vi "Tray_Search_PressIndex.vi"(0 "TrayIn":refnum<vi>, 5 "XY_DTray":cluster{"X":i32, "Y":i32}={"X"=8, "Y"=16}, 7 "Press_Arr":bool[][](array[boolean]), 9 "Record_Arr In":bool[][](array[boolean])) -> (6 "Press_Arr Out":bool[][](array[boolean]), 8 "Record_Arr Out":bool[][](array[boolean]))   [LabVIEW 2019]
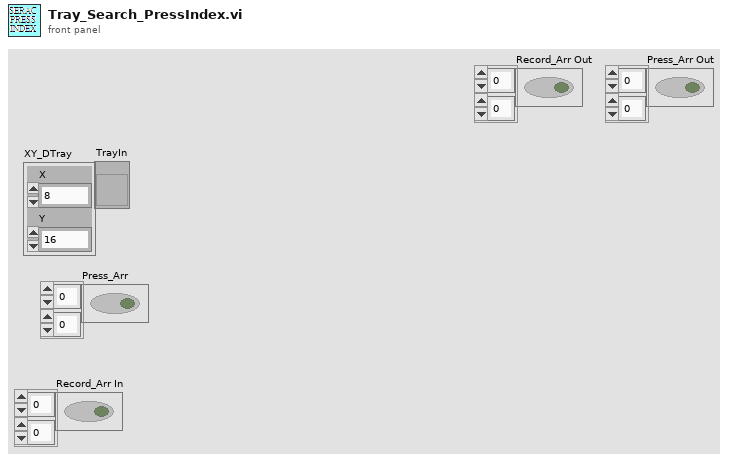
[diagram p1: front panel]
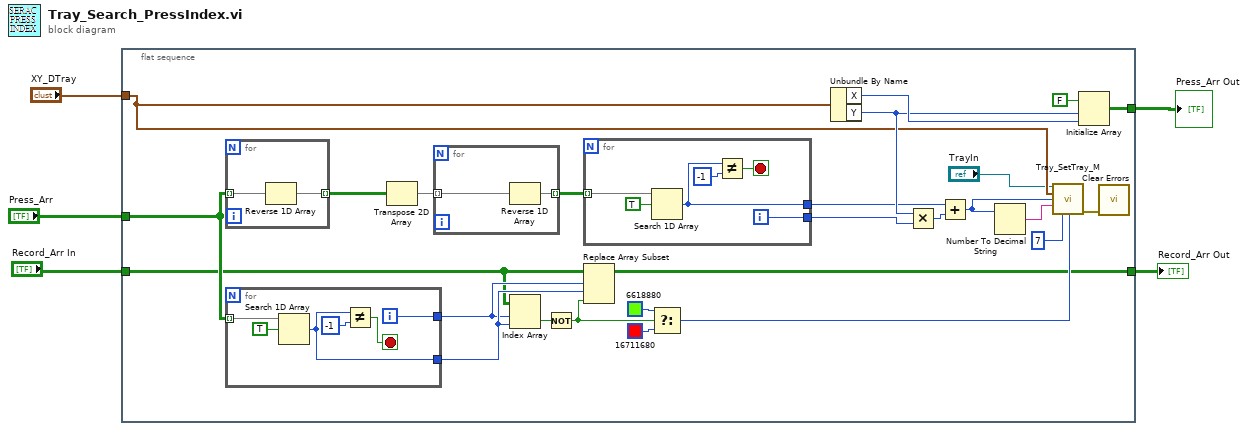
[diagram p0: block diagram]
diagram:
  n1 = flat-sequence {
    tunnel: [w26] -> w3
    tunnel: "Press_Arr" -> [w11]
    tunnel: "Record_Arr In" -> [w10]
    tunnel: "XY_DTray" -> [w9]
    tunnel: [w8] -> w1
    frame #0 {
      n2 = for {
        tunnel: [w47] -> w31 mode=indexing
        tunnel: w11 -> [w46] mode=indexing
        n3 = Reverse 1D Array(array=w46) -> (reversed array=w47:bool[])
      }
      n4 = for {
        tunnel: w11 -> [w37] mode=indexing
        tunnel: [w34] -> w12
        tunnel: [w33] -> w13
        i -> [w34]
        stop <- w35 stop-if-true
        n5 = Search 1D Array(1D array=w37, element=TRUE) -> (index of element=w33:i32)  [unwired: 1 in]
        n6 = Not Equal?(x=w33, y=-1) -> (x != y?=w35:bool)
      }
      n7 = Transpose 2D Array(2D array=w31) -> (transposed array=w30:bool[][])
      n8 = for {
        tunnel: w30 -> [w45] mode=indexing
        tunnel: [w44] -> w23 mode=indexing
        n9 = Reverse 1D Array(array=w45) -> (reversed array=w44:bool[])
      }
      n10 = Index Array(array=w10, index (row)=w12, index (col)=w13) -> (element=w18:bool)
      n11 = Not(x=w18) -> (.not. x?=w16:bool)
      n12 = for {
        tunnel: w23 -> [w43] mode=indexing
        tunnel: [w40] -> w20
        tunnel: [w39] -> w19
        i -> [w40]
        stop <- w41 stop-if-true
        n13 = Search 1D Array(1D array=w43, element=TRUE) -> (index of element=w39:i32)  [unwired: 1 in]
        n14 = Not Equal?(x=w39, y=-1) -> (x != y?=w41:bool)
      }
      n15 = Replace Array Subset(array=w10, new element=w16, index (row)=w12, index (col)=w13) -> (w8:bool[][])
      n16 = Select(t=u32 6618880 ("Color Box"), s=w16, f=u32 16711680 ("Color Box")) -> (s? t:f=w14:u32)
      n17 = Unbundle By Name(w9) -> ("X"=w22:i32, "Y"=w21:i32)
      n18 = Multiply(x=w21, y=w20) -> (x*y=w27:i32)
      n19 = Add(x=w19, y=w27) -> (x+y=w28:i32)
      n20 = Number To Decimal String(number=w28) -> (decimal integer string=w29:string)  [unwired: 1 in]
      n21 = call "Tray_SetTray_M.vi"("TrayIn"="TrayIn", "GridSize"=w9, "Index Number"=w28, "String"=w29, "Direction"=u16 7, "Color Box"=w14) -> ("error out"=w7:errorcluster)  [unwired: 9 in]
      n22 = Initialize Array(FALSE, w21, w22) -> (w26:bool[][])
      n23 = call <vilib>:"Clear Errors.vi"("error in (no error)"=w7) -> ()  [unwired: 5 in, 2 out]
    }
  }
  "Press_Arr Out" <- w3
  "Record_Arr Out" <- w1
